vi "SS Launch Subsystem.vi"(8 "error in (no error)":errorcluster, 10 "Curr Device Name":string, 11 "Data Q":refnum<queue>) -> (0 "error out":errorcluster, 1 "cmd q":T1, 2 "vi ref":refnum<vi>, 3 "Temp Ctl Class":refnum<class "Subsystem Class Temp Control.lvclass">)   [LabVIEW 2024]
uses:
  SS cluster Data Queue type.ctl
  Subsystem Class Temp Control/Subsystem Class Temp Control.lvclass
  C:/Development/rimas/RIMAS/Subsystems/Subsystem Class.lvclass
  SS typedef Cmd Queue Reference.ctl
  SS typedef cluster Instrument Command Queue Data.ctl
  Subsystem Class.lvclass/Subsystem Class.ctl
  SS Read cmd q.vi
  Subsystem Class.lvclass
  hk-channel-class/hk-channel-class/HK Item/HK Item.lvclass
panel:
  in  "error in (no error)":errorcluster
  out "error out":errorcluster
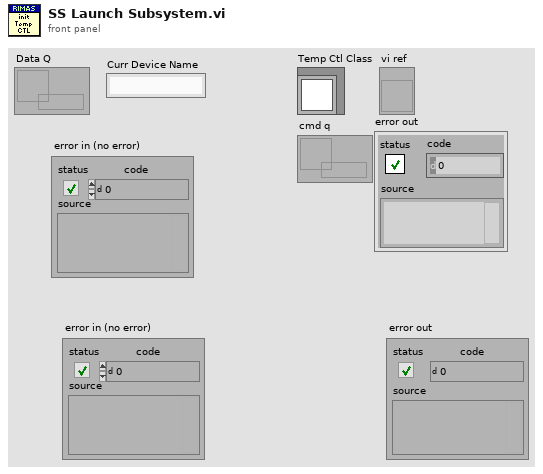
[diagram p1: front panel]
types:
  T1 = typedef "SS typedef Cmd Queue Reference.ctl" = refnum<queue>
  T2 = typedef "SS cluster Data Queue type.ctl" = cluster{"Source":string, "Type":string, "Data":variant}
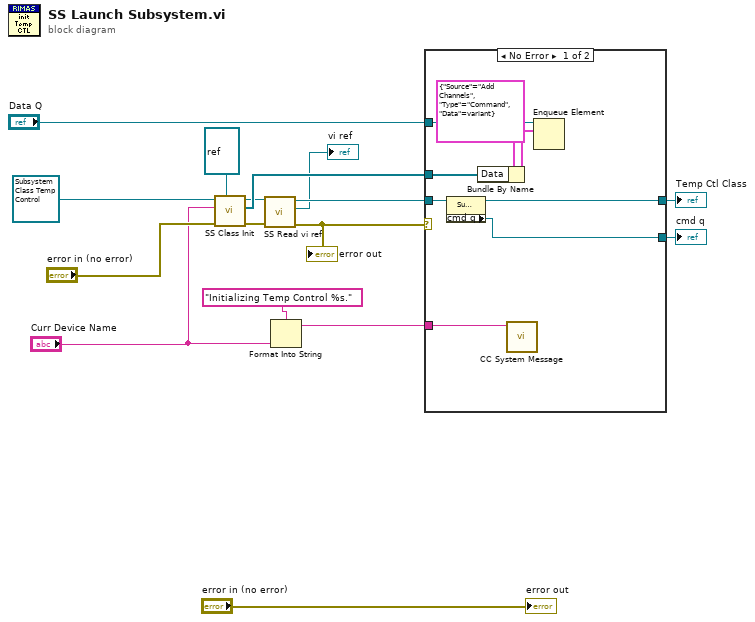
[diagram p0: block diagram]
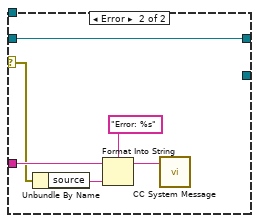
[diagram p2: hidden frame]
diagram:
  n1 = call-dynamic "SS Class Init.vi"("VI Refnum"=refnum<vi> refnum, "error in (no error)"="error in (no error)", "Device"="Curr Device Name", "Subsystem Class Temp Control in"=refnum<class "Subsystem Class Temp Control.lvclass"> refnum ("Subsystem Class Temp Control.lvclass")) -> ("error out"=w15:errorcluster, "Channel List"=w11:refnum<class "HK Item.lvclass">[], "Subsystem Class Temp Control out"=w9:refnum<class "Subsystem Class Temp Control.lvclass">)  [unwired: 5 in]
  n2 = call "SS Read vi ref.vi"("error in (no error)"=w15, "Subsystem Class in"=w9) -> ("error out"=w8:errorcluster, "vi ref"=→"vi ref":refnum<vi>, "Subsystem Class out"=w12:refnum<class "Subsystem Class Temp Control.lvclass">)  [unwired: 7 in]
  "error out" <- w8
  n3 = Format Into String(format string="Initializing Temp Control %s.", "Curr Device Name") -> (resulting string=w13:string)  [unwired: 2 in, 1 out]
  n4 = case shown="No Error" w8 {
    selector: w8 -> [_ w28]
    tunnel: w13 -> [w19 w29]
    tunnel: w12 -> [w24 w25]
    tunnel: w11 -> [w21 _]
    tunnel: "Data Q" -> [w23 _]
    tunnel: [w18 w25] -> w4
    tunnel: [w17 _] -> w3
    frame No Error {
      n5 = property class="Subsystem Class Temp Control.lv"(reference=w24) -> (reference out=w18:refnum<class "Subsystem Class Temp Control.lvclass">, "cmd q"=w17:T1)  [unwired: 1 in, 1 out]
      n6 = Bundle By Name(cluster=T2 {"Source"="Add Channels", "Type"="Command", "Data"=variant} ("element"), "Data"=w21) -> (w20:T2)
      n7 = call "CC System Message.vi"("Message"=w19) -> ()  [unwired: 10 in, 1 out]
      n8 = Enqueue Element(queue=w23, element=w20) -> ()  [unwired: 2 in, 3 out]
    }
    frame Error {
      n9 = Unbundle By Name(w28) -> ("source"=w27:string)
      n10 = Format Into String(format string="Error: %s", initial string=w29, w27) -> (resulting string=w26:string)  [unwired: 1 in, 1 out]
      n11 = call "CC System Message.vi"("Message"=w26) -> ()  [unwired: 10 in, 1 out]
    }
  }
  "Temp Ctl Class" <- w4
  "cmd q" <- w3
  "error out" <- "error in (no error)"
